vi "ex_Read Properties.vi"(4 "Ignore Errors":bool, 5 "Control Data":T3(array[cluster]) {"Ctl Type" items=["Control", "Constant", "Title", "Tag", "Tag(String)", "DDT Control", "Tag (Numeric)"]}, 6 "viref Configuration Dialog":refnum<vi>, 7 "viref Instance":refnum<vi>) -> (0 "viref Configuration Dialog out":refnum<vi>, 1 "Output Cluster":T1)   [LabVIEW 2017]
doc: "Performs the initial step for the Property Page of an Express VI. These tasks include making sure the items specified in the Control Data array have the correct labels and match the appropriate items in both the Express VI and the property page, checking the values of all the items in the Express VI, and returning the refnums an other information that will be needed later in the property page."
uses:
  <vilib>/express/express shared/propPagePersistenceType.ctl
  <vilib>/express/express shared/propPageData.ctl
panel:
  in  "Configuration Dialog":string="Configuration Dialog."
  in  "Instance.":string="Instance."
  in  "Couldn't find control/constant on the":string="\nCouldn't find control/constant on the "
  in  "Control Label:":string="**\nError in prop page construction:\nControl Label: "
  out "Both":bool[](array[boolean])
  out "Configuration\nDialog\n(all false)":bool[](array[boolean])
  out "Instance\n(Instance name t, \nall else f)":bool[](array[boolean])
  out "Control Types":i32[](array[numeric])=[48, 10, 10, 10, 64, 33, 10, 3] format="%x"
  out "PropPage Ctl Refs":refnum<vi>[](array[refnum])
  out "Instance Ctl Refs":refnum<vi>[](array[refnum])
  in  "Configuration Dialog Ctl Label":string
  in  "Instance Ctl Label":string
  in  "Ctl Type":u16(ring)=3 items=["Number", "String", "Boolean", "Constant"]
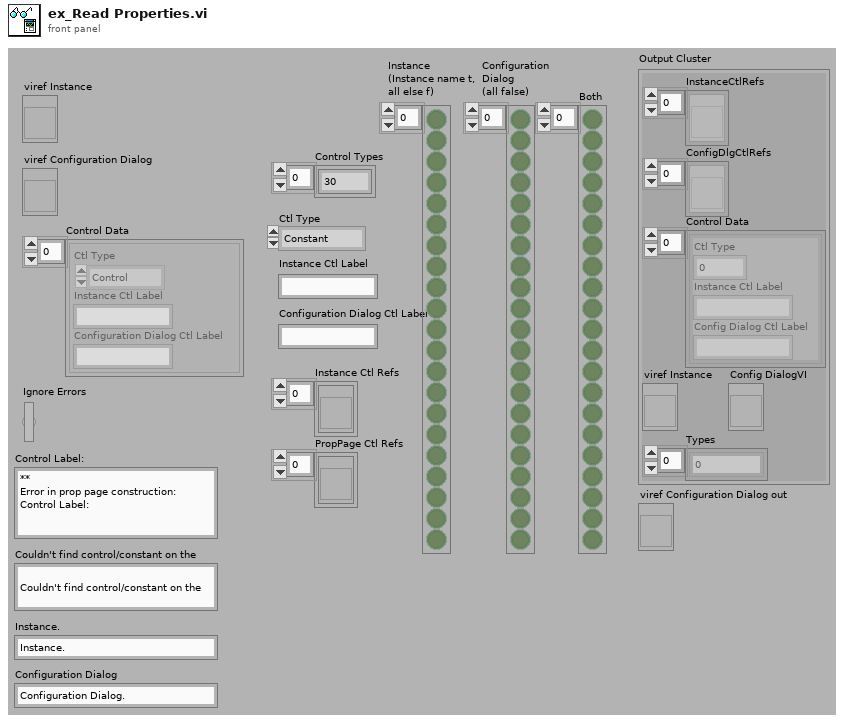
[diagram p1: front panel]
types:
  T1 = typedef "propPageData.ctl" = cluster{"InstanceCtlRefs":refnum<vi>[], "ConfigDlgCtlRefs":refnum<vi>[], "Control Data":cluster{"Ctl Type":u16, "Instance Ctl Label":string, "Config Dialog Ctl Label":string}[], "viref Instance":refnum<vi>, "Types":i32[], "Config DialogVI":refnum<vi>}
  T2 = typedef "propPagePersistenceType.ctl" = u16
  T3 = cluster{"Ctl Type":T2, "Instance Ctl Label":string, "Configuration Dialog Ctl Label":string}[]
  T4 = cluster{"Ctl Type":T2, "Express VI Ctl Label":string, "PropPage Ctl Label":string}[]
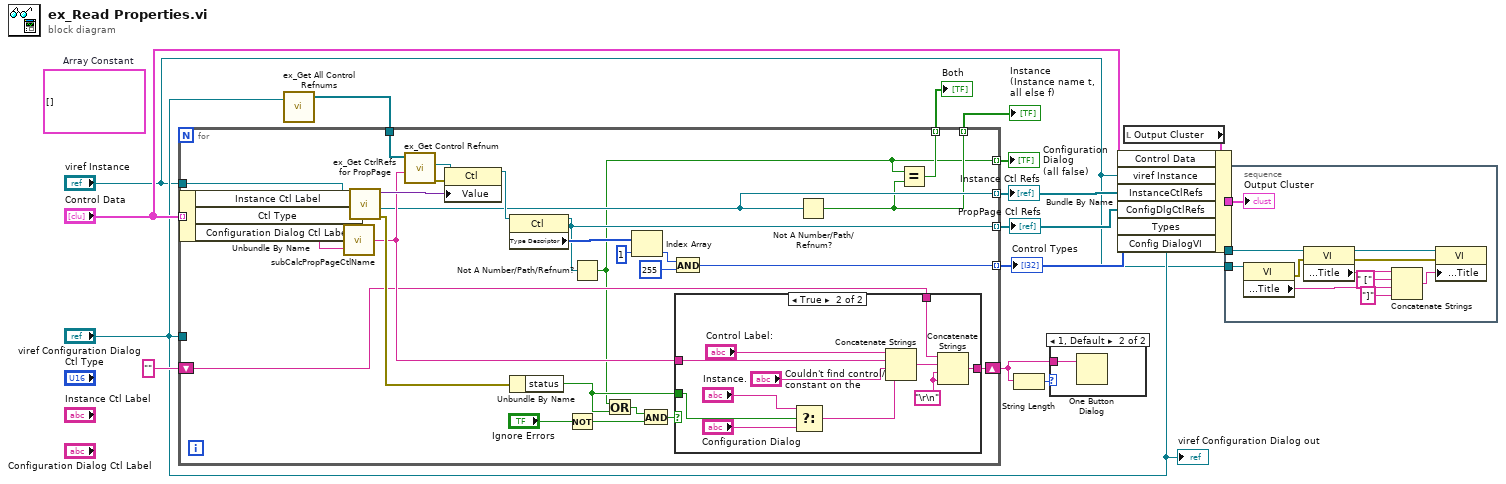
[diagram p0: block diagram]
diagram:
  (unwired) T4 []  # Array Constant
  n1 = call <vilib>:"ex_Get All Control Refnums.vi"("viref Express VI"="viref Configuration Dialog") -> ("All Controls[]"=w14:refnum<vi>[])  [unwired: 2 in, 1 out]
  n2 = for {
    tunnel: "Control Data" -> [w44] mode=indexing
    tunnel: "viref Instance" -> [w37]
    tunnel: "viref Configuration Dialog" -> [_]
    tunnel: [w21] -> w5 mode=indexing
    tunnel: [w22] -> w6 mode=indexing
    tunnel: [w41] -> w15 mode=indexing
    tunnel: w14 -> [w28]
    shift-right: [w24] -> w12
    shift-left: "" -> [w25]
    tunnel: [w20] -> w10 mode=indexing
    tunnel: [w18] -> w9 mode=indexing
    tunnel: [w19] -> w8 mode=indexing
    n3 = Unbundle By Name(w44) -> ("Instance Ctl Label"=w36:string, "Ctl Type"=w17:T2, "Configuration Dialog Ctl Label"=w16:string)
    n4 = call <vilib>:"subCalcPropPageCtlName.vi"("Property Page Ctl Label"=w16, "Express VI Ctl Label"=w36) -> ("Prop Ctl Name"=w27:string)
    n5 = call <vilib>:"ex_Get CtrlRefs for PropPage.vi"("Ctl Type"=w17, "Object Name"=w36, "Express VI"=w37) -> ("error out"=w31:errorcluster, "Output Reference"=w22:refnum<vi>, "Value"=w35:variant)  [unwired: 6 in]
    n6 = call <vilib>:"ex_Get Control Refnum.vi"("Name"=w27, "Controls[]"=w28) -> ("error out"=w23:errorcluster, "Ctl Refnum"=w26:refnum<vi>)  [unwired: 8 in]
    n7 = property class="Ctl"(reference=w26, error in=w23, "Value"=w35) -> (reference out=w39:refnum<vi>)  [unwired: 1 out]
    n8 = property class="Ctl"(reference=w39) -> (reference out=w21:refnum<vi>, "Type Descriptor"=w38:i16[])  [unwired: 1 in, 1 out]
    n9 = Unbundle By Name(w31) -> ("status"=w29:bool)
    n10 = Not(x="Ignore Errors") -> (.not. x?=w33:bool)
    n11 = Not A Number/Path/Refnum?(number/path/refnum=w21) -> (NaN/Path/Refnum?=w18:bool)
    n12 = Or(x=w18, y=w29) -> (x .or. y?=w30:bool)
    n13 = Index Array(array=w38, index=1 ("Index")) -> (element=w40:i16)
    n14 = And(x=w30, y=w33) -> (x .and. y?=w32:bool)
    n15 = And(x=w40, y=255) -> (x .and. y?=w41:i32)
    n16 = case shown="True" w32 {
      tunnel: w27 -> [_ w55]
      tunnel: w29 -> [_ w50]
      tunnel: w25 -> [w45 w48]
      tunnel: [w45 w47] -> w24
      frame False {
      }
      frame True {
        w46 = "\r\n"
        n17 = Select(t="Instance.", s=w50, f="Configuration Dialog") -> (s? t:f=w53:string)
        n18 = Concatenate Strings("Control Label:", w55, "Couldn't find control/constant on the", w53) -> (w49:string)
        n19 = Concatenate Strings(w48, w49, w46, w46) -> (w47:string)
      }
    }
    n20 = Not A Number/Path/Refnum?(number/path/refnum=w22) -> (NaN/Path/Refnum?=w20:bool)
    n21 = Equal?(x=w18, y=w20) -> (x = y?=w19:bool)
  }
  "Instance Ctl Refs" <- w6
  "PropPage Ctl Refs" <- w5
  "Control Types" <- w15
  "Instance\n(Instance name t, \nall else f)" <- w10
  "Configuration\nDialog\n(all false)" <- w9
  "Both" <- w8
  n22 = String Length(string=w12) -> (length=w13:i32)
  n23 = case shown="1, Default" w13 {
    tunnel: w12 -> [_ w57]
    frame 0 {
    }
    frame 1, Default {
      n24 = One Button Dialog(message=w57) -> ()  [unwired: 1 in, 1 out]
    }
  }
  n25 = local read "Output Cluster"() -> (w7:T1)
  n26 = Bundle By Name(cluster=w7, "Control Data"="Control Data", "viref Instance"="viref Instance", "InstanceCtlRefs"=w6, "ConfigDlgCtlRefs"=w5, "Types"=w15, "Config DialogVI"="viref Configuration Dialog") -> (w1:T1)
  n27 = stacked-sequence {
    tunnel: "viref Configuration Dialog" -> [w62]
    tunnel: "viref Instance" -> [w59]
    tunnel: w1 -> [w58]
    frame #0 {
      n28 = property class="VI"(reference=w59) -> (error out=w60:errorcluster, "Front Panel Window:Title"=w61:string)  [unwired: 1 in, 1 out]
      n29 = property class="VI"(reference=w62, error in=w60) -> (reference out=w68:refnum<vi>, error out=w63:errorcluster, "Front Panel Window:Title"=w67:string)
      n30 = Concatenate Strings(w67, " [" ("string"), w61, "]" ("string")) -> (w64:string)
      n31 = property class="VI"(reference=w68, error in=w63, "Front Panel Window:Title"=w64) -> ()  [unwired: 2 out]
      "Output Cluster" <- w58
    }
  }
  "viref Configuration Dialog out" <- "viref Configuration Dialog"
